vi "Lectura de temperatura(SubVI).vi"(11 "file path (use dialog)":path) -> (0 "error out":errorcluster, 2 "error out 2":errorcluster, 3 "Array":dbl[](array[numeric]))   [LabVIEW 2021]
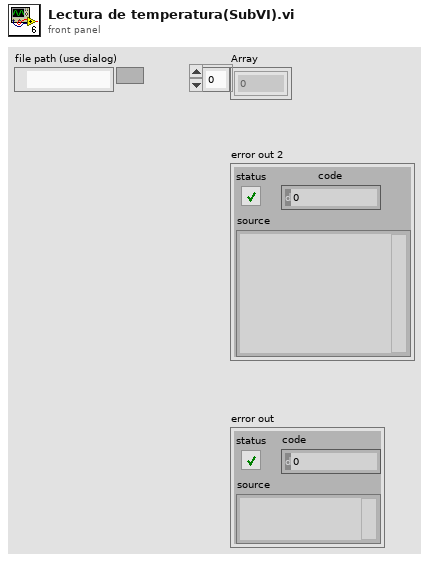
[diagram p1: front panel]
types:
  T1 = enum16{"open", "replace", "create", "open or create", "replace or create", "replace or create with confirmation"}
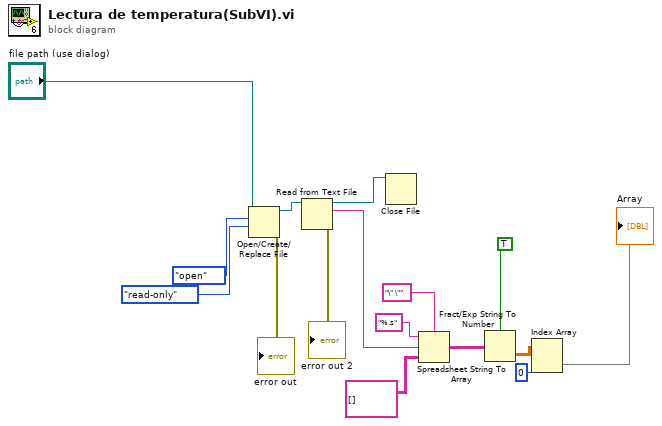
[diagram p0: block diagram]
diagram:
  n1 = Open/Create/Replace File(file path (use dialog)="file path (use dialog)", operation (0:open)=T1."open", access (0:read/write)=enum16{"read/write", "read-only", "write-only"}."read-only") -> (refnum out=w10:refnum<file>, error out=→"error out":errorcluster)  [unwired: 3 in, 1 out]
  n2 = Read from Text File(file (use dialog)=w10) -> (refnum out=w9:refnum<file>, text=w5:string, error out=→"error out 2":errorcluster)  [unwired: 3 in, 1 out]
  n3 = Close File(refnum=w9) -> ()  [unwired: 1 in, 2 out]
  n4 = Spreadsheet String To Array(delimiter (Tab)="\" \"", format string="%.s", spreadsheet string=w5, array type (2D Dbl)=string[][] []) -> (array=w3:string[][])
  n5 = Fract/Exp String To Number(use system decimal point (T)=TRUE, string=w3) -> (number=w13:dbl[][])  [unwired: 2 in, 1 out]
  n6 = Index Array(array=w13, index (col)=0 ("disabled index (col)")) -> (element=→"Array":dbl[])  [unwired: 1 in]
